vi "Write terms to map.vi"(10 "Terminals In":T1[](array[typedef]), 11 "Block Diagram in":T2) -> (3 "Block Diagram Out":T2)   [LabVIEW 2025]
uses:
  Controls/bd.ctl
  Classes/Node/Node.lvclass
  Controls/wire.ctl
  Controls/Terminal.ctl
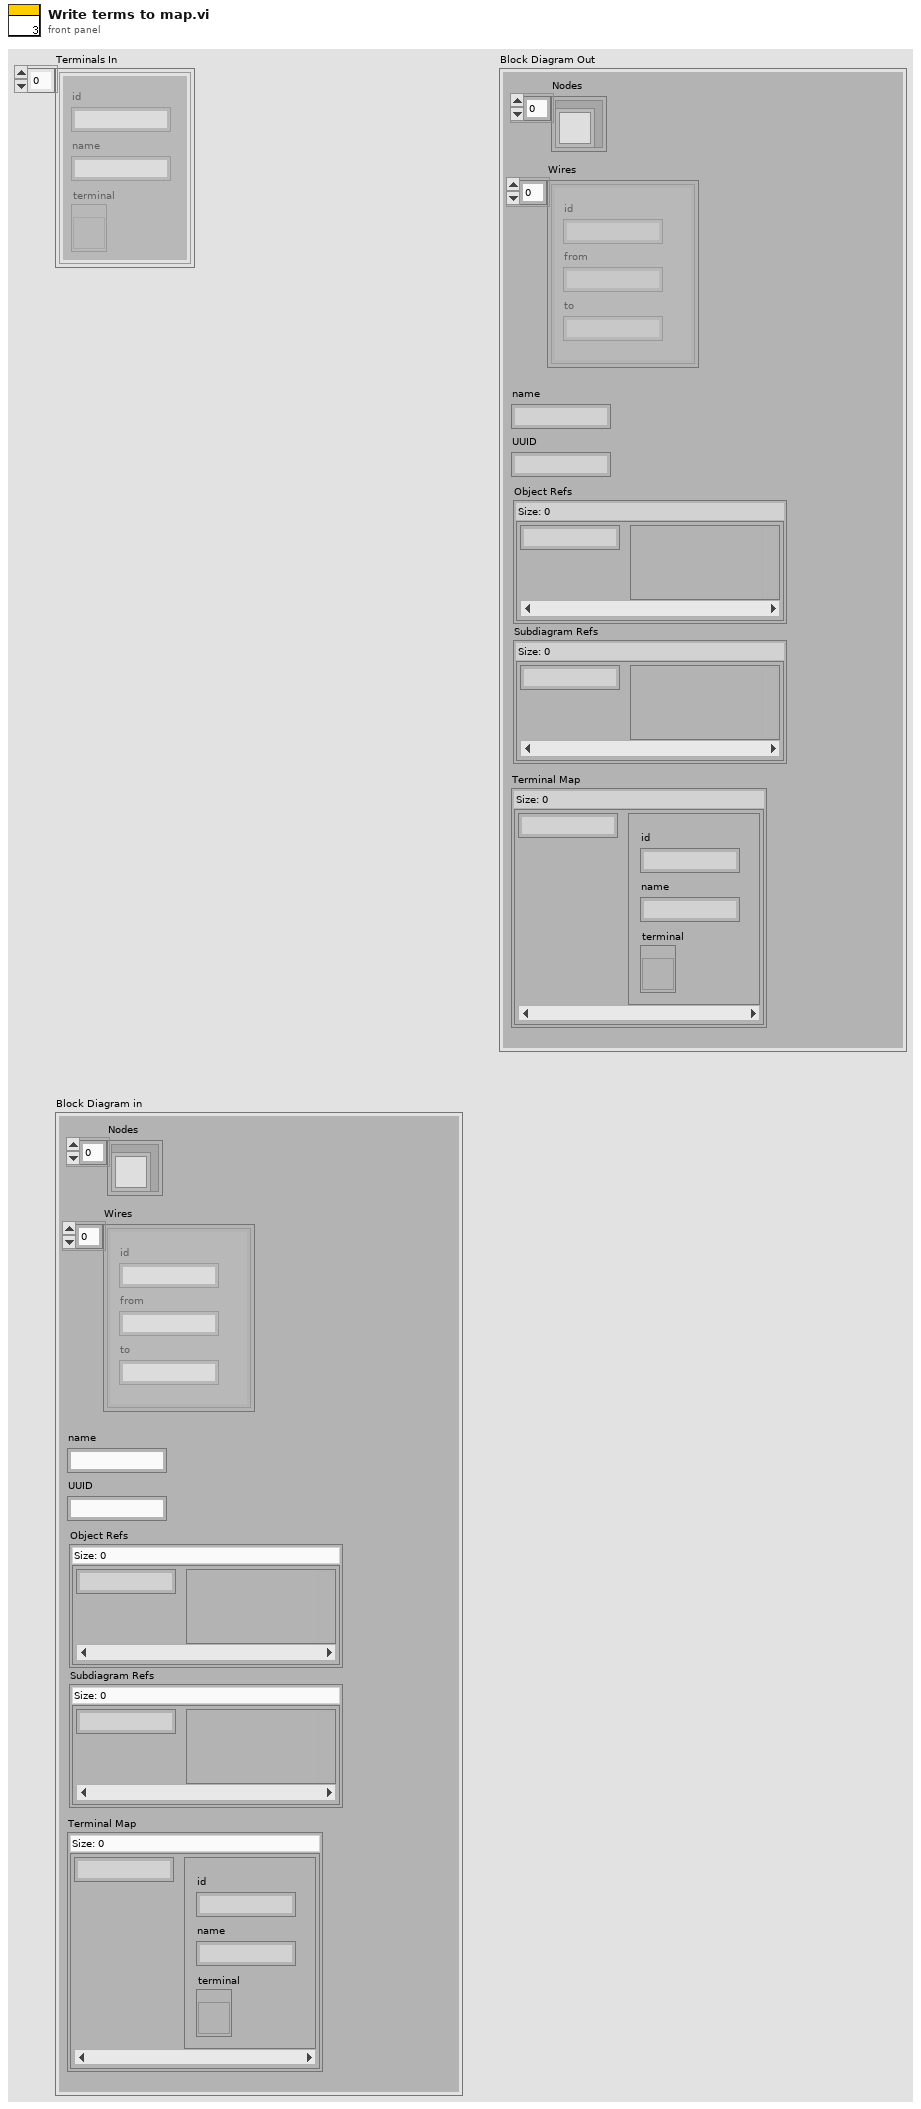
[diagram p1: front panel]
types:
  T1 = typedef "Terminal.ctl" = cluster{"id":string, "name":string, "terminal":refnum<vi>}
  T2 = typedef "bd.ctl" = cluster{"Nodes":refnum<class "Node.lvclass">[], "Wires":T3[], "name":string, "UUID":string, "Object Refs":map{string, variant}, "Subdiagram Refs":map{string, variant}, "Terminal Map":map{string, T1}}
  T3 = typedef "wire.ctl" = cluster{"id":string, "from":string, "to":string}
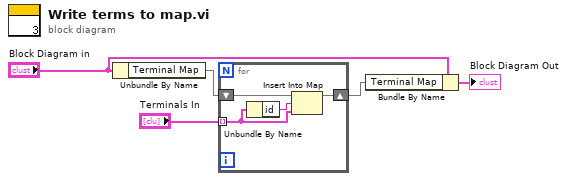
[diagram p0: block diagram]
diagram:
  n1 = Unbundle By Name("Block Diagram in") -> ("Terminal Map"=w2:map{string, T1})
  n2 = for {
    shift-right: [w8] -> w4
    shift-left: w2 -> [w9]
    tunnel: "Terminals In" -> [w7] mode=indexing
    n3 = Unbundle By Name(w7) -> ("id"=w6:string)
    n4 = Insert Into Map(map in=w9, key=w6, value=w7) -> (map out=w8:map{string, T1})  [unwired: 2 out]
  }
  n5 = Bundle By Name(cluster="Block Diagram in", "Terminal Map"=w4) -> (→"Block Diagram Out":T2)
